vi "SandBox - Set As Top Level VI.vi"   [LabVIEW 2016]
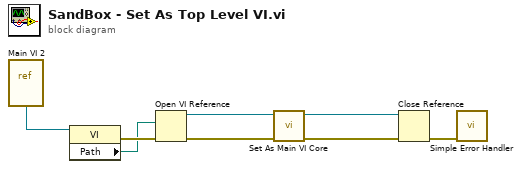
[diagram p0: block diagram]
diagram:
  n1 = vi-ref "Main VI 2.vi"() -> (w8:refnum<vi>)
  n2 = property class="VI"(reference=w8) -> (error out=w7:errorcluster, "Path"=w2:path)  [unwired: 1 in, 1 out]
  n3 = Open VI Reference(vi path=w2, error in (no error)=w7) -> (vi reference=w6:refnum<vi>, error out=w5:errorcluster)  [unwired: 4 in]
  n4 = call "Set As Main VI Core.vi"("error in (no error)"=w5, "Calling VI Ref in"=w6) -> ("error out"=w3:errorcluster, "Calling VI Ref out"=w4:refnum<vi>)  [unwired: 8 in]
  n5 = Close Reference(reference=w4, error in (no error)=w3) -> (error out=w1:errorcluster)
  n6 = call <vilib>:"Simple Error Handler.vi"("error in (no error)"=w1) -> ()  [unwired: 4 in, 5 out]
